vi "RSZVB Define Group Of Measured Ports.vi"(6 "First Port (1)":i32=1, 7 "Last Port (1)":i32=1, 8 "error in (no error)":errorcluster {"code" format="%.0x"}, 9 "Group (1)":i32=1, 10 "Channel (1)":i32=1, 11 "VISA session":refnum<visa-resource-name>) -> (0 "error out":errorcluster {"code" format="%.0x"}, 3 "dup VISA session":refnum<visa-resource-name>)   [LabVIEW 2011]
doc: "This VI defines a group of measured ports numbered <Group> containing a continuous range of logical ports <First Port> and <Last Port>.\n\nRemote-control command(s):\nSOURce<Ch>:GROup<group_no>"
uses:
  _utility/RSZVB Global Data.vi
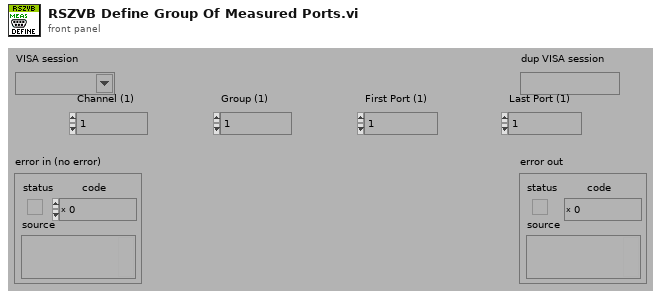
[diagram p1: front panel]
types:
  T1 = cluster{"Error Checking (T: On)":bool, "Installed Options":string[], "Data Valid?":bool, "Ports":i32, "Model":string[], "Option Checking (T: On)":bool}[]
  T2 = cluster{"Error Checking (T: On)":bool, "Installed Options":string[], "Data Valid?":bool, "Ports":i32, "Model":string[], "Option Checking (T: On)":bool}
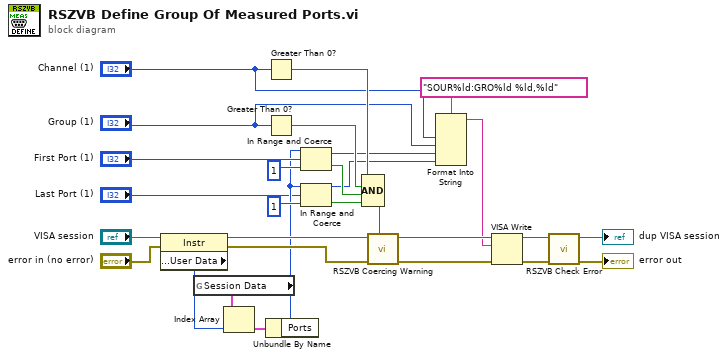
[diagram p0: block diagram]
diagram:
  n1 = property class="Instr"(reference="VISA session", error in="error in (no error)") -> (reference out=w11:refnum<visa-resource-name>, error out=w12:errorcluster, "General Settings:User Data"=w13:u32)
  n2 = global read "RSZVB Global Data.vi" "Session Data"() -> (w14:T1)
  n3 = Index Array(array=w14, index=w13) -> (element=w15:T2)
  n4 = Greater Than 0?(x="Channel (1)") -> (x > 0?=w16:bool)
  n5 = Greater Than 0?(x="Group (1)") -> (x > 0?=w17:bool)
  n6 = Unbundle By Name(w15) -> ("Ports"=w6:i32)
  n7 = In Range and Coerce(upper limit=w6, x="First Port (1)", lower limit=1) -> (coerced(x)=w2:i32, In Range?=w23:bool)
  n8 = In Range and Coerce(upper limit=w6, x="Last Port (1)", lower limit=1) -> (coerced(x)=w1:i32, In Range?=w7:bool)
  n9 = Compound Arithmetic op=AND(w16, w17, w23, w7) -> (w22:bool)
  n10 = call "RSZVB Coercing Warning.vi"("In Range?"=w22, "error in (no error)"=w12, "VISA session"=w11) -> ("error out"=w26:errorcluster, "dup VISA session"=w27:refnum<visa-resource-name>)  [unwired: 7 in]
  n11 = Format Into String(format string="SOUR%ld:GRO%ld %ld,%ld", "Channel (1)", "Group (1)", w2, w1) -> (resulting string=w21:string)  [unwired: 2 in, 1 out]
  n12 = VISA Write(VISA resource name=w27, write buffer=w21, error in (no error)=w26) -> (VISA resource name out=w24:refnum<visa-resource-name>, error out=w25:errorcluster)  [unwired: 1 out]
  n13 = call "RSZVB Check Error.vi"("error in (no error)"=w25, "VISA session"=w24) -> ("error out"=→"error out":errorcluster, "dup VISA session"=→"dup VISA session":refnum<visa-resource-name>)  [unwired: 8 in]
